vi "testWrist.vi"() -> ()   [LabVIEW 2015]
panel:
  in  "Select Servo":string(combo)="Servo 1"
  in  "angle":i32
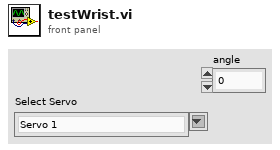
[diagram p1: front panel]
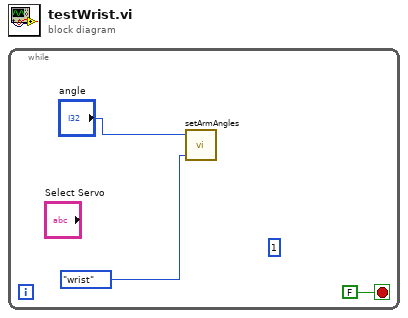
[diagram p0: block diagram]
diagram:
  n1 = while {
    stop <- FALSE stop-if-true
    (unwired) u8 1 ("Controller Daisy Chain Position (1 - 4)")
    n2 = call "setArmAngles.vi"("Enum"=enum16{"shoulder", "elbow", "wrist"}."wrist", "angle"="angle") -> ()  [unwired: 2 in]
  }
